vi "temp chart with pid sim start.vi"(1 "stop":bool, 7 "Control Parameters":T4={"Setpoint"=60.0, "Control bandwidth"=10.0, "Settle bandwidth"=1.0, "Integral time"=10.0, "Int\non"=TRUE, "Derivative time"=0.5, "Der\non"=TRUE, "Settle time"=60.0} {"Settle time" format="%.2f"; "Derivative time" format="%.2f"; "Integral time" format="%.2f"; "Settle bandwidth" format="%.2f"; "Control bandwidth" format="%.2f"; "Setpoint" format="%.2f"}, 11 "error in":errorcluster, 12 "Manual Override":bool) -> (8 "Temp":dbl format="%.2f", 10 "Time in Settle Band":dbl format="%.2f", 14 "settled":bool, 15 "error out":errorcluster)   [LabVIEW 2016]
doc: "This vi records and plots the temperature of a 10 kOhm thermsitor using an Agilent 34405A as the measurment device.\n\nIt sets the power to the heater resistor using the NI ELVIS Variable DC, and measures the power using DAQ analog in.\n\nIt uses a PID feedback algorithm to obtain the desired setpoint.\n\nPaul K Dixon\nPhysics 350\nCSUSB Physics"
uses:
  typedefs/control parameters.ctl
  typedefs/status indicator.ctl
  typedefs/scale control.ctl
  <vilib>/Utility/miscctls.llb/LVPointTypeDef.ctl
  components/therm sim/therm sim kernel/globals/therm sim globals.vi
panel:
  in  "milliseconds to wait":u32(slide)=500 scale=0.0..500.0
  in  "convection":dbl(slide) scale=0.0..10.0
  in  "Scale Control":T1
  in  "Power Control":dbl(slide) scale=0.0..1.0
  out "range indicators":T2={"In control band"=FALSE, "In settle band"=FALSE, "under range"=TRUE, "over range"=FALSE}
  out "Power":dbl=0.754407202908737 format="%.2f"
  out "Setpoint":dbl=50.0 format="%.2f"
  out "Temperature History":T3(graph)={"temp out"=29.702811899974034, 50.0, 50.5, 49.5, 50.1, 49.9, 50.508814405817475}
  # "SIM PID Temperature Controller"
  # "1.0"
  # "Norm\nPower\nscale"
  # "0.5"
  # "0.0"
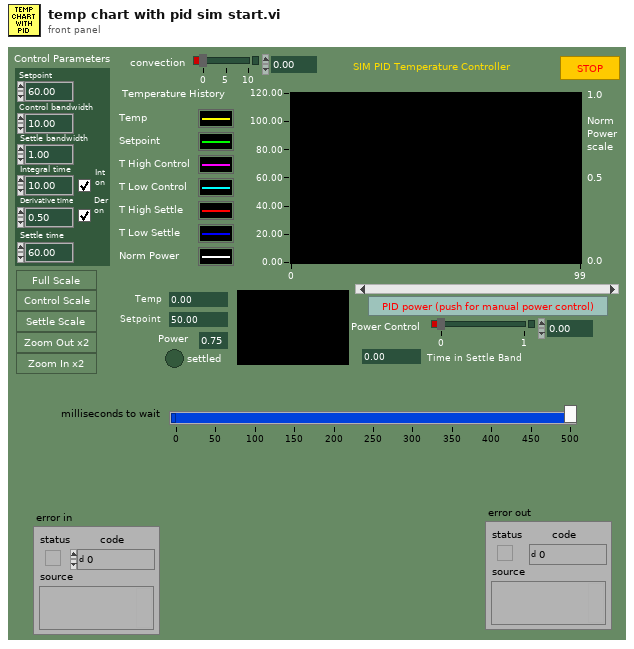
[diagram p1: front panel]
types:
  T1 = typedef "scale control.ctl" = cluster{"Full Scale":bool, "Control Scale":bool, "Settle Scale":bool, "Zoom Out":bool, "Zoom In":bool}
  T2 = typedef "status indicator.ctl" = cluster{"In control band":bool, "In settle band":bool, "under range":bool, "over range":bool}
  T3 = cluster{"temp out":dbl, dbl, dbl, dbl, dbl, dbl, dbl}
  T4 = typedef "control parameters.ctl" = cluster{"Setpoint":dbl, "Control bandwidth":dbl, "Settle bandwidth":dbl, "Integral time":dbl, "Int\non":bool, "Derivative time":dbl, "Der\non":bool, "Settle time":dbl}
  T5 = typedef "LVPointTypeDef.ctl" = cluster{"Horizontal":i16, "Vertical":i16}
  T6 = cluster{"[0]":refnum<vi>, "[1]":refnum<vi>, "[2]":refnum<vi>, "[3]":refnum<vi>}
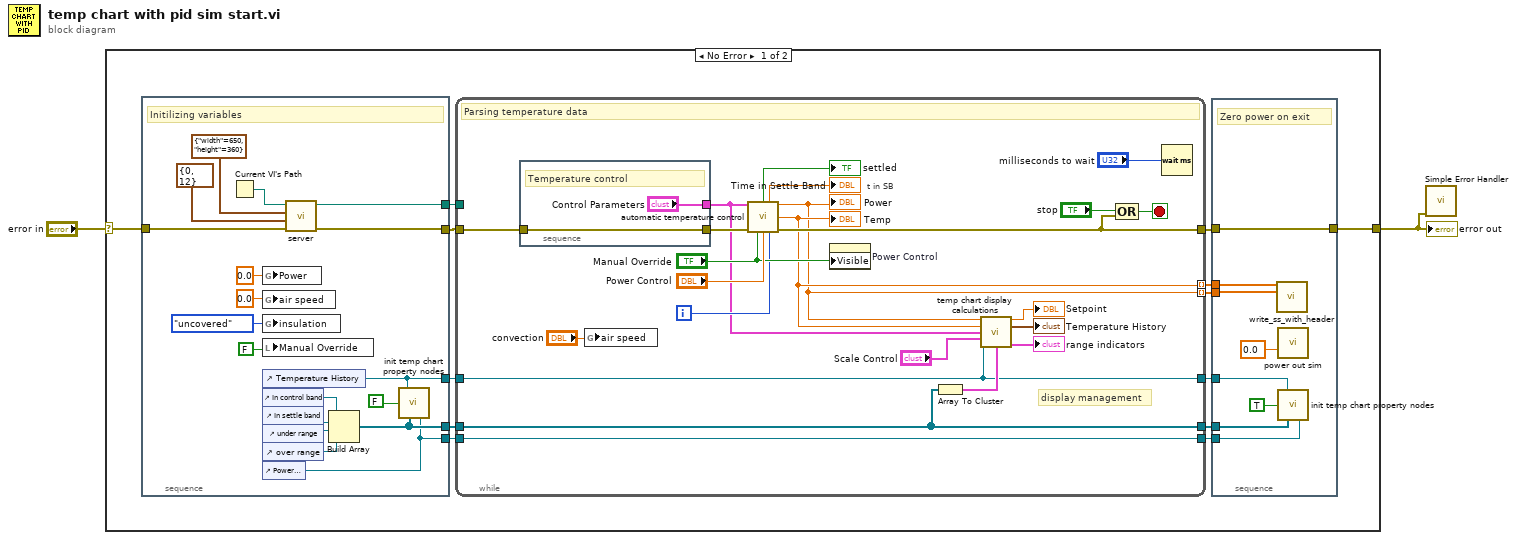
[diagram p0: block diagram]
diagram:
  n1 = case shown="No Error" "error in" {
    selector: "error in" -> [w13 w67]
    tunnel: [w14 w67] -> w1
    frame No Error {
      n2 = stacked-sequence {
        tunnel: w13 -> [w54]
        tunnel: [w61] -> w12
        tunnel: [w62] -> w11
        tunnel: [w59] -> w7
        tunnel: [w53] -> w6
        tunnel: [w50] -> w5
        frame #0 {
          # "Initilizing variables"
          n3 = Current VI's Path() -> (path=w51:path)
          n4 = global write "therm sim globals.vi" "Power"(0.0 ("Power")) -> ()
          n5 = global write "therm sim globals.vi" "air speed"(0.0 ("air speed")) -> ()
          n6 = global write "therm sim globals.vi" "insulation"(enum16{"uncovered", "covered"}."uncovered" ("insulation")) -> ()
          n7 = local write "Manual Override"(FALSE ("Manual Override")) -> ()
          n8 = control-ref of="Temperature History"() -> (w62:refnum<vi>)
          n9 = control-ref of="In control band"() -> (w63:refnum<vi>)
          n10 = control-ref of="In settle band"() -> (w64:refnum<vi>)
          n11 = control-ref of="under range"() -> (w65:refnum<vi>)
          n12 = control-ref of="over range"() -> (w66:refnum<vi>)
          n13 = control-ref of="Power Control"() -> (w59:refnum<vi>)
          n14 = call "server.vi"("error in (no error)"=w54, "Origin"=T5 {"Horizontal"=0, "Vertical"=12}, "Window Dimensions"=cluster{"width":i16, "height":i16} {"width"=650, "height"=360}, "path in"=w51) -> ("error out"=w53:errorcluster, "path out"=w50:path)  [unwired: 6 in]
          n15 = Build Array(w63, w64, w65, w66) -> (w61:refnum<vi>[])
          n16 = call "init temp chart property nodes.vi"("Temperature History"=w62, "Power control visible"=FALSE ("Visible"), "range indicators"=w61, "Power Control"=w59) -> ()  [unwired: 2 in, 10 out]
        }
      }
      n17 = while {
        tunnel: w7 -> [w23]
        tunnel: [w23] -> w8
        tunnel: [w24] -> w9
        tunnel: [w25] -> w10
        tunnel: w11 -> [w24]
        tunnel: w12 -> [w25]
        tunnel: w6 -> [w27]
        tunnel: [w20] -> w15
        tunnel: w5 -> [_]
        tunnel: [w18] -> w4 mode=indexing
        tunnel: [w17] -> w3 mode=indexing
        i -> [w22]
        stop <- w29 stop-if-true
        # "display management"
        # "t in SB"
        # "Parsing temperature data"
        n18 = stacked-sequence {
          tunnel: ["Control Parameters"] -> w16
          tunnel: w27 -> [w39]
          tunnel: [w39] -> w28
          frame #0 {
            # "Temperature control"
          }
        }
        n19 = global write "therm sim globals.vi" "air speed"("convection") -> ()
        n20 = call "automatic temperature control.vi"("Control Parameters"=w16, "error in"=w28, "Manual Override"="Manual Override", "Normalized Power In (0-1)"="Power Control", "index (0=init)"=w22) -> ("settled"=→"settled":bool, "time in settle band"=→"Time in Settle Band":dbl, "power meas (0-1)"=w17:dbl, "temp meas"=w18:dbl, "error out"=w20:errorcluster)  [unwired: 2 in, 4 out]
        "Temp" <- w18
        "Power" <- w17
        n21 = property on="Power Control" class="Slide (strict)"("Visible"="Manual Override") -> ()  [unwired: 2 in, 2 out]
        n22 = Array To Cluster(array=w25) -> (cluster=w26:T6)
        n23 = call "temp chart display calculations.vi"("power in (0-1)"=w17, "temp in"=w18, "Control Parameters"=w16, "Scale Control In"="Scale Control", "Temp History in"=w24, "range indicator refs"=w26) -> ("Setpoint out"=→"Setpoint":dbl, "Temperature History out"=→"Temperature History":T3, "range indicators out"=→"range indicators":T2)  [unwired: 3 in, 4 out]
        n24 = Compound Arithmetic op=OR("stop", w20) -> (w29:bool)
        n25 = Wait (ms)(milliseconds to wait="milliseconds to wait") -> ()  [unwired: 1 out]
      }
      n26 = stacked-sequence {
        tunnel: [w48] -> w14
        tunnel: w15 -> [w48]
        tunnel: w10 -> [w46]
        tunnel: w8 -> [w44]
        tunnel: w9 -> [w43]
        tunnel: w4 -> [w42]
        tunnel: w3 -> [w41]
        frame #0 {
          # "Zero power on exit"
          n27 = call "write_ss_with_header.vi"("temp"=w42, "power"=w41) -> ()  [unwired: 14 in]
          n28 = call "power out sim.vi"("Normalized Power (0-1)"=0.0 ("Normalized\n Power (0-1)")) -> ()  [unwired: 2 in, 13 out]
          n29 = call "init temp chart property nodes.vi"("Temperature History"=w43, "Power control visible"=TRUE ("Visible"), "range indicators"=w46, "Power Control"=w44) -> ()  [unwired: 2 in, 10 out]
        }
      }
    }
    frame Error {
    }
  }
  "error out" <- w1
  n30 = call <vilib>:"Simple Error Handler.vi"("error in (no error)"=w1) -> ()  [unwired: 4 in, 5 out]
